vi "ConfigSaveAS.vi"(10 "Get All Control Values Variant":cluster{"Name":string, "Variant Data":variant}[](array[cluster]), 11 "String in":refnum<vi>) -> ()   [LabVIEW 2014]
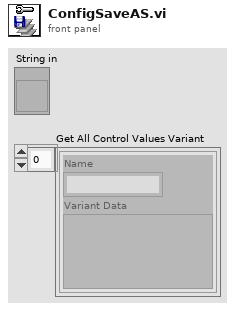
[diagram p1: front panel]
types:
  T1 = enum16{"open", "open or create", "create or replace", "create", "open (read only)"}
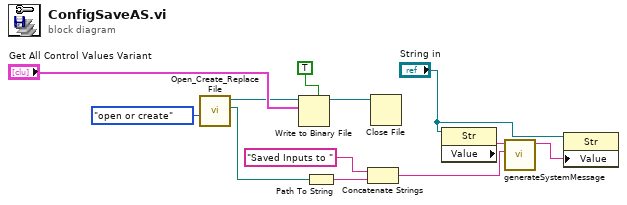
[diagram p0: block diagram]
diagram:
  n1 = call <vilib>:"Open_Create_Replace File.vi"("function (open:0)"=T1."open or create") -> ("new file path"=w12:path, "refnum"=w3:refnum<file>)  [unwired: 7 in, 2 out]
  n2 = Write to Binary File(file (use dialog)=w3, data="Get All Control Values Variant", 5:TRUE ("header (F)")) -> (refnum out=w4:refnum<file>)  [unwired: 3 in, 2 out]
  n3 = Path To String(path=w12) -> (string=w9:string)
  n4 = Concatenate Strings("Saved Inputs to " ("string"), w9) -> (w11:string)
  n5 = Close File(refnum=w4) -> ()  [unwired: 1 in, 2 out]
  n6 = property on="Property Node" class="Str"(reference="String in") -> ("Value"=w8:string)  [unwired: 1 in, 2 out]
  n7 = call "generateSystemMessage.vi"("New Message"=w11, "Old Message"=w8) -> ("System Message Output"=w7:string)  [unwired: 9 in]
  n8 = property on="Property Node" class="Str"(reference="String in", "Value"=w7) -> ()  [unwired: 1 in, 2 out]
